vi "test_error_indicator.vi"() -> ()   [LabVIEW 2019]
panel:
  in  "value3":dbl[](array[numeric])=[4.0, 11.0, 4.0, 9.0, 13.0]
  in  "value2":dbl=10.0
  in  "lolo2":dbl=-10.0
  in  "hihi2":dbl=10.0
  out "steps":i32=11
  in  "wait":u32=1000 caption="ms"
  in  "value1":dbl=10.0
  in  "stop":bool
  in  "lo":dbl=-5.0
  in  "lolo":dbl=-10.0
  in  "hihi":dbl=10.0
  in  "hi":dbl=5.0
  # "error & warning"
  # "error only"
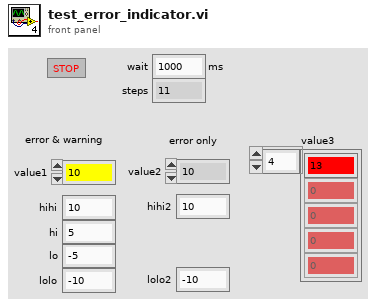
[diagram p1: front panel]
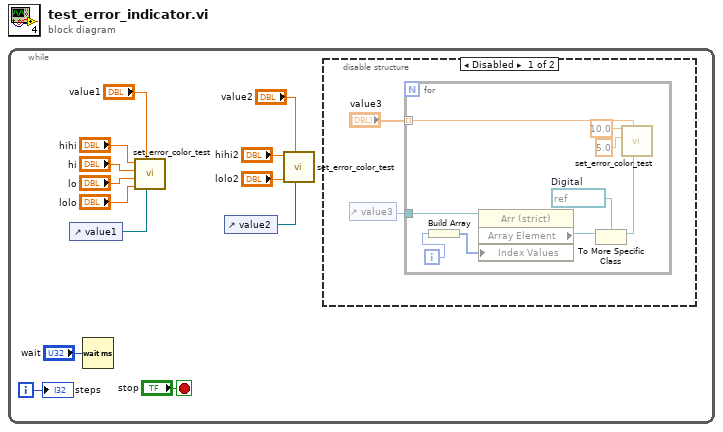
[diagram p0: block diagram]
diagram:
  n1 = while {
    i -> [w11]
    stop <- "stop" stop-if-true
    n2 = control-ref of="value1"() -> (w2:refnum<vi>)
    n3 = Wait (ms)(milliseconds to wait="wait") -> ()  [unwired: 1 out]
    n4 = call "set_error_color_test.vi"("value_ref"=w2, "value"="value1", "lolo"="lolo", "lo"="lo", "hi"="hi", "hihi"="hihi") -> ()  [unwired: 6 in]
    n5 = control-ref of="value2"() -> (w1:refnum<vi>)
    n6 = call "set_error_color_test.vi"("value_ref"=w1, "value"="value2", "lolo"="lolo2", "hihi"="hihi2") -> ()  [unwired: 8 in]
    n7 = disable-structure shown="Disabled" {
      frame Disabled {
        n8 = control-ref of="value3"() -> (w14:refnum<vi>)
        n9 = for {
          tunnel: "value3" -> [w24] mode=indexing
          tunnel: w14 -> [w23]
          i -> [w18]
          w20 = refnum<vi> refnum  # Digital
          n10 = Build Array(w18) -> (w19:i32[])
          n11 = property class="Arr (strict)"(reference=w23, "Index Values"=w19) -> ("Array Element"=w22:refnum<vi>)  [unwired: 1 in, 2 out]
          n12 = To More Specific Class(target class=w20, reference=w22) -> (specific class reference=w21:refnum<vi>)  [unwired: 1 in, 1 out]
          n13 = call "set_error_color_test.vi"("value_ref"=w21, "value"=w24, "hi"=5.0, "hihi"=10.0) -> ()  [unwired: 8 in]
        }
      }
      frame Enabled {
      }
    }
    "steps" <- w11
  }
